vi "Insert Log.vi"(8 "error in (no error)":errorcluster, 10 "log":string[](array[string]), 11 "Logger Normal in":refnum<class "Logger Normal.lvclass">) -> (0 "error out":errorcluster, 3 "Logger Normal out":refnum<class "Logger Normal.lvclass">)   [LabVIEW 2020, in "Logger Normal.lvlib" / "Logger Normal.lvclass"]
uses:
  Logger Normal.lvclass
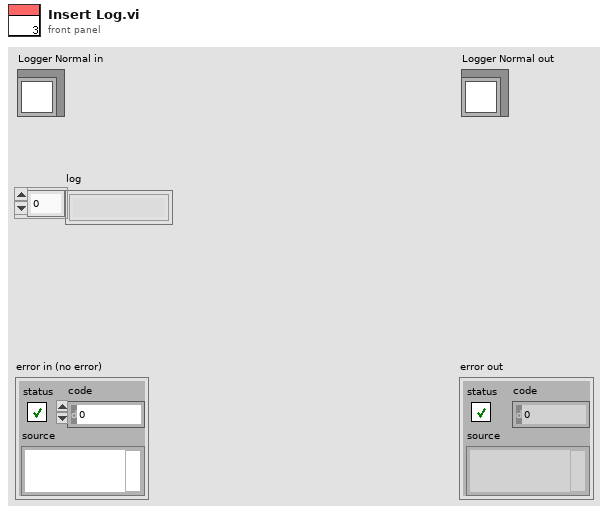
[diagram p1: front panel]
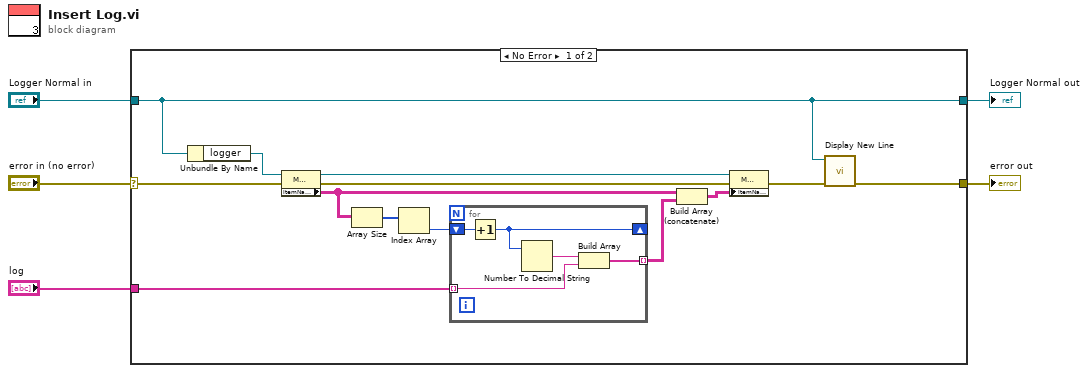
[diagram p0: block diagram]
diagram:
  n1 = case shown="No Error" "error in (no error)" {
    selector: "error in (no error)" -> [w18 w25]
    tunnel: [w7 w25] -> w4
    tunnel: [w6 w24] -> w2
    tunnel: "Logger Normal in" -> [w6 w24]
    tunnel: "log" -> [w10 _]
    frame No Error {
      n2 = Unbundle By Name(w6) -> ("logger"=w17:refnum<vi>)
      n3 = property class="MCListbox (strict)"(reference=w17, error in=w18) -> (reference out=w15:refnum<vi>, error out=w16:errorcluster, "ItemNames"=w13:string[][])
      n4 = Array Size(array=w13) -> (size(s)=w12:i32[])
      n5 = Index Array(array=w12) -> (element=w11:i32)  [unwired: 1 in]
      n6 = for {
        tunnel: w10 -> [w20] mode=indexing
        shift-right: [w22] -> _
        shift-left: w11 -> [w23]
        tunnel: [w19] -> w9 mode=indexing
        n7 = Increment(x=w23) -> (x+1=w22:i32)
        n8 = Number To Decimal String(number=w22) -> (decimal integer string=w21:string)  [unwired: 1 in]
        n9 = Build Array(w21, w20) -> (w19:string[])
      }
      n10 = Build Array (concatenate)(w13, w9) -> (w14:string[][])
      n11 = property class="MCListbox (strict)"(reference=w15, error in=w16, "ItemNames"=w14) -> (error out=w8:errorcluster)  [unwired: 1 out]
      n12 = call "Display New Line.vi"("error in (no error)"=w8, "Logger Normal in"=w6) -> ("error out"=w7:errorcluster)  [unwired: 8 in, 1 out]
    }
    frame Error {
    }
  }
  "error out" <- w4
  "Logger Normal out" <- w2
